vi "Module - Home Page.vi"() -> ()   [LabVIEW 2020]
uses:
  Control/State - eFGV.ctl
panel:
  out "Site Name":string="RUMAH KUNJAN (8.19kWp)"
  out "SI-01-FREQ":dbl caption="FREQ" format="%.0f Hz"
  out "SI-01-L3":dbl caption="L3" format="%.0f V"
  out "SI-01-L2":dbl caption="L2" format="%.0f V"
  out "SI-01-L1":dbl caption="L1" format="%.0f V"
  out "SI-01-PAC":dbl caption="Pac" format="%.0f W"
  out "BANK-02-TEMP":dbl caption="T_bat" format="%#_g °C"
  out "BANK-02-IDC":dbl caption="I_bat" format="%#_g A"
  out "BANK-02-VDC":dbl caption="V_bat" format="%#_g V"
  out "BANK-02-SOC":dbl caption="SOC" format="%#_g %"
  out "SB-02-B-IAC":dbl caption="B.Idc" format="%.0f A"
  out "SB-02-B-VAC":dbl caption="B.Vdc" format="%.0f V"
  out "SB-02-A-IAC":dbl caption="A.Idc" format="%.0f A"
  out "SB-02-A-VAC":dbl caption="A.Vdc" format="%.0f V"
  out "SB-02-PAC":dbl caption="Pac" format="%#_g W"
  out "PM-01-FREQ":dbl caption="Freq" format="%.0f Hz"
  out "PM-01-IAC":dbl caption="Iac" format="%.0f A"
  out "PM-01-VAC":dbl caption="Vac" format="%.0f V"
  out "PM-01-PAC":dbl caption="Pac" format="%.0f W"
  out "SI-M-FREQ":dbl caption="FREQ" format="%.0f Hz"
  out "SI-M-L3":dbl caption="L3" format="%.0f V"
  out "SI-M-L2":dbl caption="L2" format="%.0f V"
  out "SI-M-L1":dbl caption="L1" format="%.0f V"
  out "SI-M-PAC":dbl caption="Pac" format="%.0f W"
  out "BANK-01-TEMP":dbl caption="T_bat" format="%#_g °C"
  out "BANK-01-IDC":dbl caption="I_bat" format="%#_g A"
  out "BANK-01-VDC":dbl caption="V_bat" format="%#_g V"
  out "BANK-01-SOC":dbl caption="SOC" format="%#_g %"
  out "SB-01-B-IAC":dbl caption="B.Idc" format="%.0f A"
  out "SB-01-B-VAC":dbl caption="B.Vdc" format="%.0f V"
  out "SB-01-A-IAC":dbl caption="A.Idc" format="%.0f A"
  out "SB-01-A-VAC":dbl caption="A.Vdc" format="%.0f V"
  out "SB-01-PAC":dbl caption="Pac" format="%.0f W"
  # "SB-01"
  # "SB-02"
  # "BANK-1"
  # "BANK-2"
  # "SI-M"
  # "SI-01"
  # "PM-01"
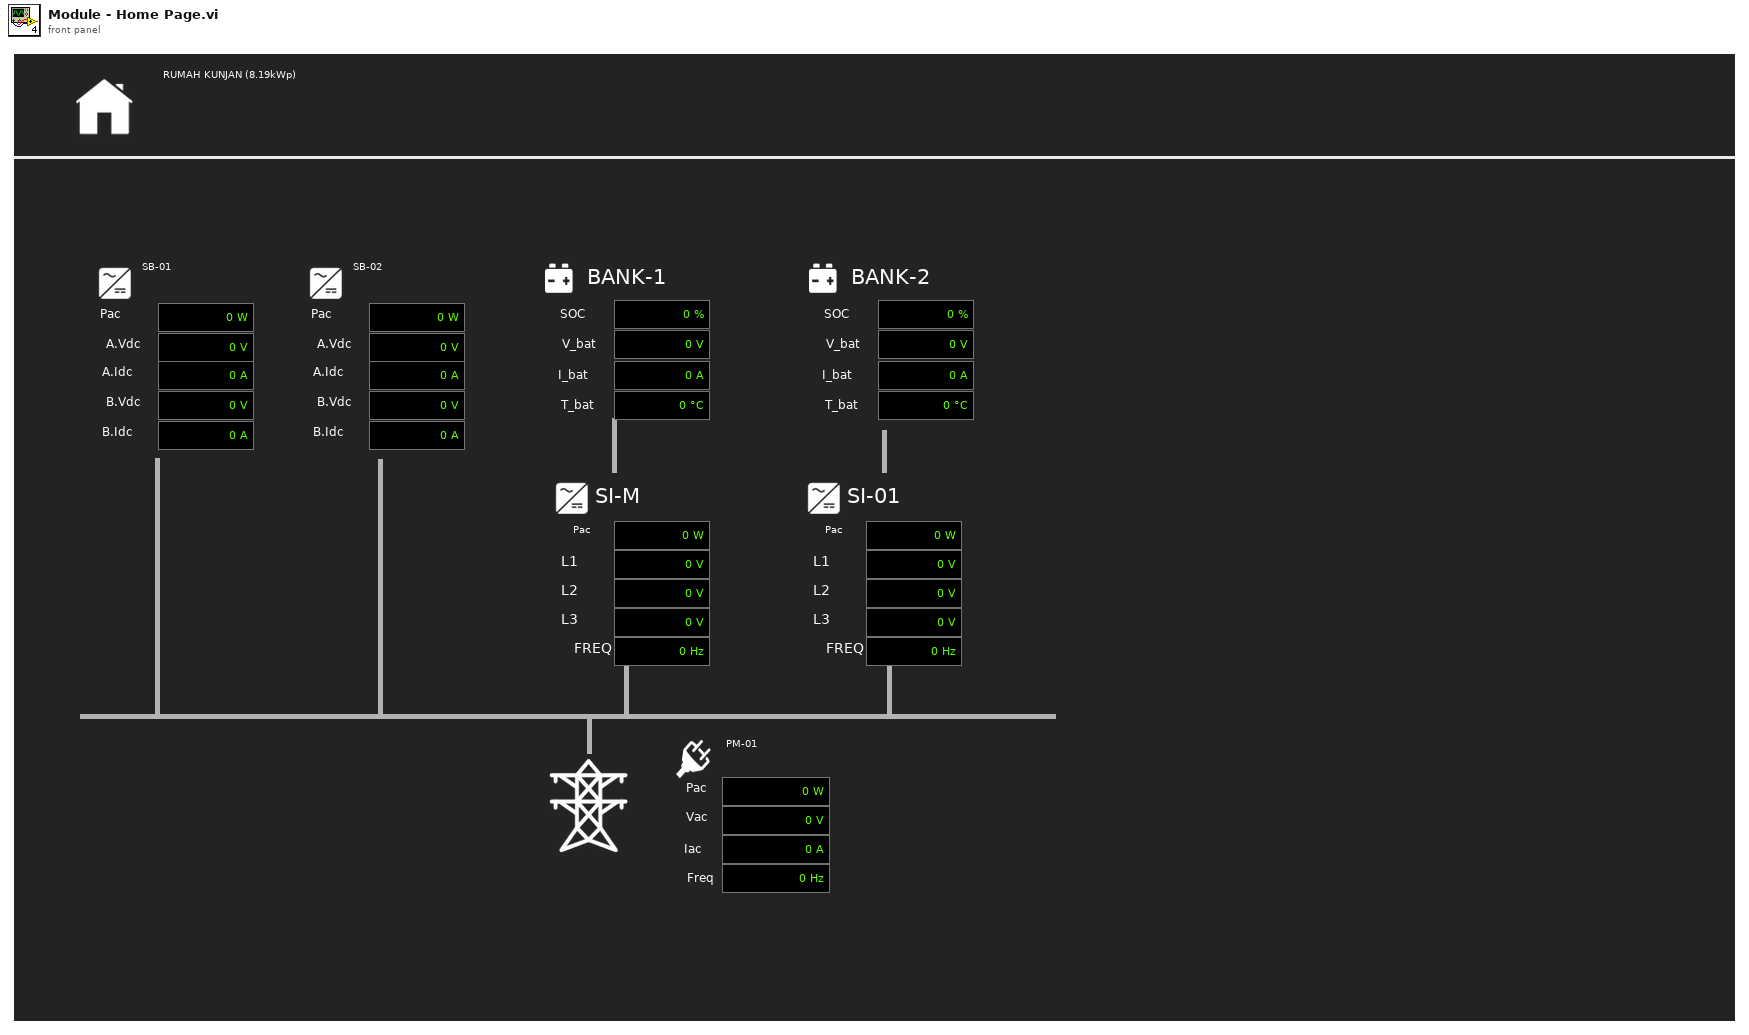
[diagram p1: front panel]
types:
  T1 = typedef "State - eFGV.ctl" = enum16{"Init", "Read", "Write", "Close"}
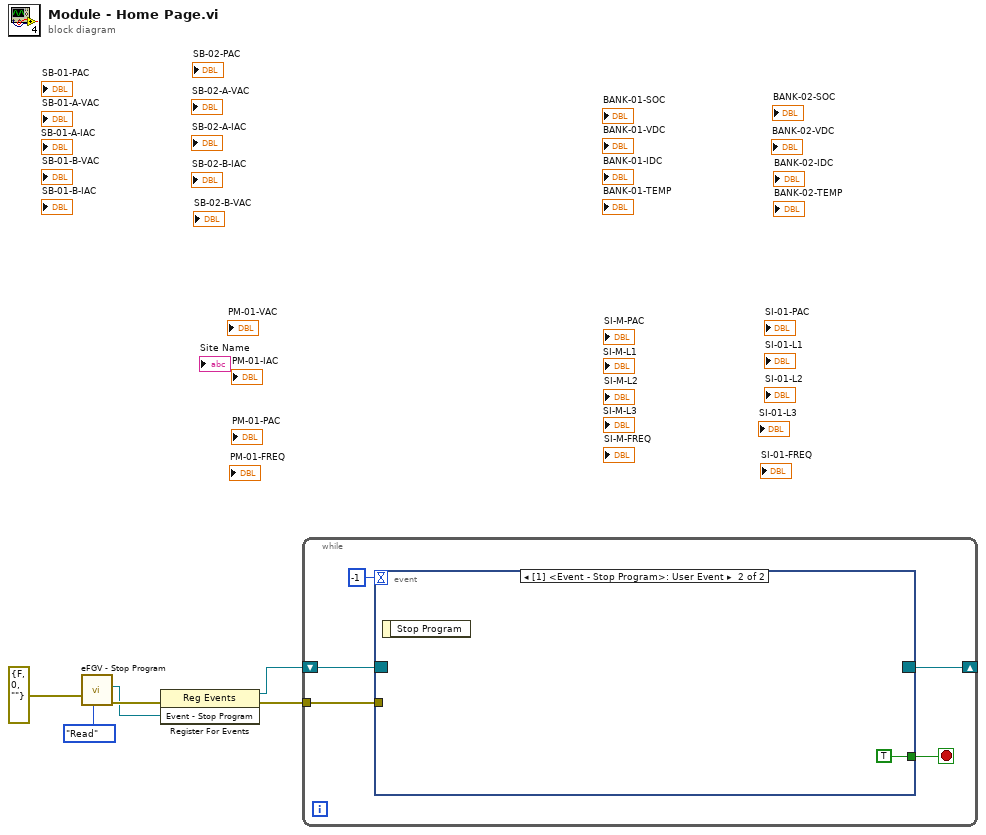
[diagram p0: block diagram]
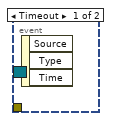
[diagram p2: hidden frame]
diagram:
  n1 = call "eFGV - Stop Program.vi"("State - eFGV"=State_-_eFGV."Read", "error in (no error)"=errorcluster {"status"=FALSE, "code"=0, "source"=""}) -> ("error out"=w5:errorcluster, "Event - Stop Program"=w4:refnum<user-event>)  [unwired: 8 in]
  n2 = register-events(error in=w5, w4) -> (reference out=w1:refnum<event-registration>, error out=w6:errorcluster)  [unwired: 1 in]
  n3 = while {
    tunnel: w6 -> [w10]
    shift-right: [w9] -> _
    shift-left: w1 -> [w11]
    stop <- w8 stop-if-true
    n4 = event shown="[1] <Event - Stop Program>: User Event" {
      selector: w11 -> [_ _]
      dyn-events: [_ _] -> w9
      timeout: -1 -> [_ _]
      tunnel: w10 -> [_ _]
      tunnel: [_ TRUE] -> w8
      event Timeout {
        n5 = event-data() -> ()  [unwired: 1 in, 3 out]
      }
      event User Event {
        n6 = event-data() -> ()  [unwired: 1 in, 1 out]
      }
    }
  }
